vi "SaveFile.vi"(6 "Logging file refnum in":refnum<file>, 7 "Threshold Exceeded?":bool, 8 "Error in":errorcluster, 9 "Sound format":T2, 10 "Filtered Data":waveform(dbl)[](array[waveform]), 11 "Sound file refnum in":T1) -> (0 "Error out":errorcluster, 3 "Sound file refnum out":T1, 4 "Logging file refnum out":refnum<file>)   [LabVIEW 2019]
uses:
  <vilib>/sound2/lvsound2.llb/Sound File Refnum.ctl
  <vilib>/sound2/lvsound2.llb/Sound File Write Open.vi
  <vilib>/sound2/lvsound2.llb/Sound File Write (DBL).vi
  <vilib>/sound2/lvsound2.llb/Sound Data Format.ctl
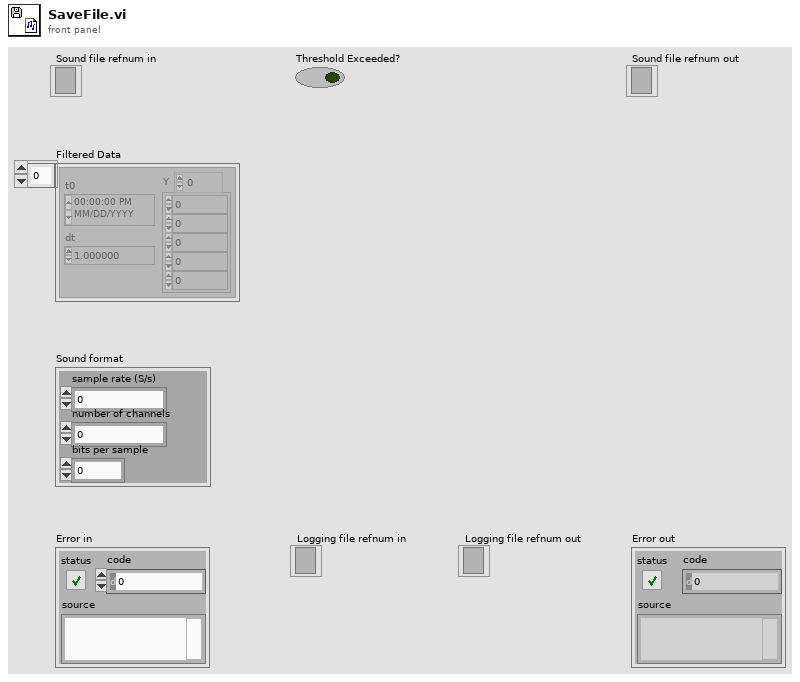
[diagram p1: front panel]
types:
  T1 = typedef "Sound File Refnum.ctl" = refnum<file>
  T2 = typedef "Sound Data Format.ctl" = cluster{"sample rate (S/s)":dbl, "number of channels":i32, "bits per sample":i32}
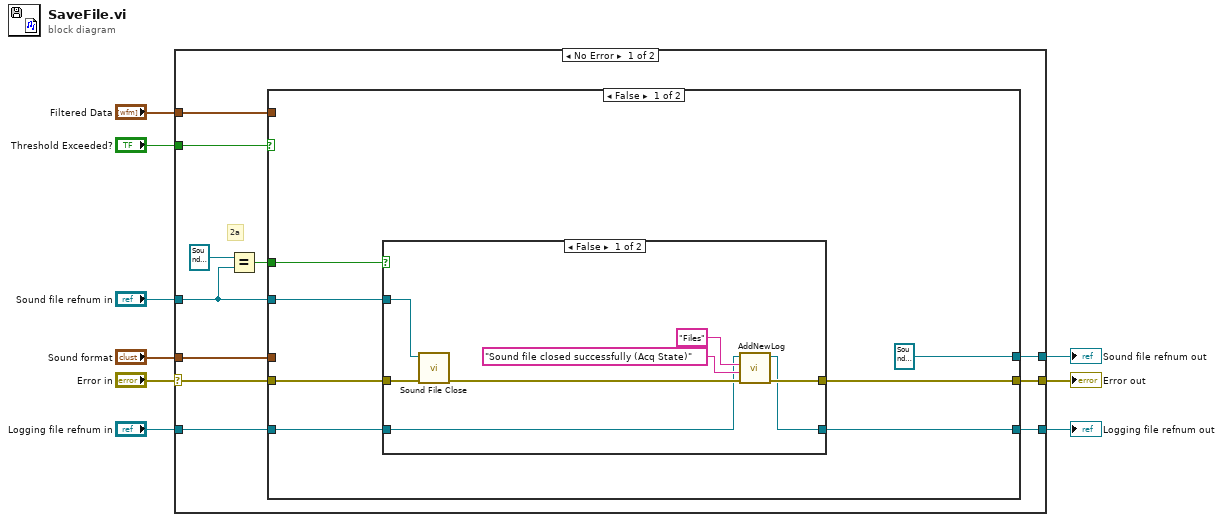
[diagram p0: block diagram]
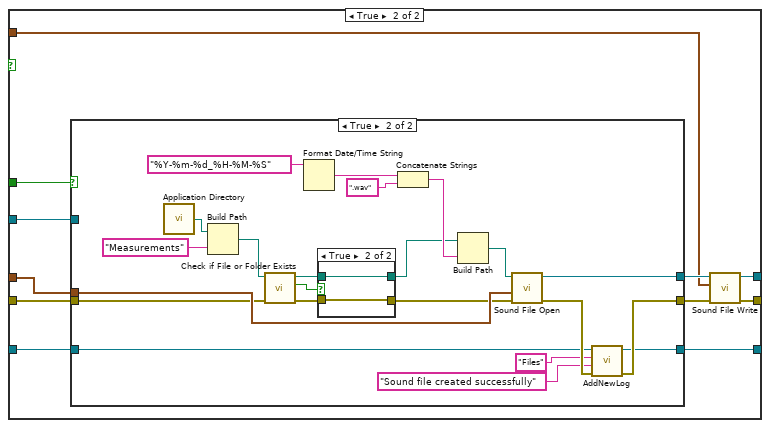
[diagram p3: hidden frame]
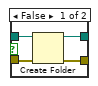
[diagram p5: hidden frame]
diagram:
  n1 = case shown="No Error" "Error in" {
    selector: "Error in" -> [w12 w82]
    tunnel: "Threshold Exceeded?" -> [w20 _]
    tunnel: "Filtered Data" -> [w19 _]
    tunnel: "Sound format" -> [w18 _]
    tunnel: [w17 w82] -> w6
    tunnel: [w16 w81] -> w5
    tunnel: "Sound file refnum in" -> [w14 w81]
    tunnel: "Logging file refnum in" -> [w11 w80]
    tunnel: [w10 w80] -> w1
    frame No Error {
      # "2a"
      n2 = Equal?(x=T1 refnum ("sound file refnum out"), y=w14) -> (x = y?=w13:bool)
      n3 = case shown="False" w20 {
        tunnel: [w25 w46] -> w17
        tunnel: w18 -> [_ w45]
        tunnel: w19 -> [_ w44]
        tunnel: w12 -> [w27 w43]
        tunnel: [T1 refnum ("sound file refnum out") w42] -> w16
        tunnel: w14 -> [w26 w40]
        tunnel: w13 -> [w23 w41]
        tunnel: w11 -> [w22 w39]
        tunnel: [w21 w38] -> w10
        frame False {
          n4 = case shown="False" w23 {
            tunnel: w27 -> [w35 w37]
            tunnel: w26 -> [w34 _]
            tunnel: [w30 w37] -> w25
            tunnel: w22 -> [w29 w36]
            tunnel: [w28 w36] -> w21
            frame False {
              n5 = call <vilib>:"Sound File Close.vi"("error in (no error)"=w35, "sound file refnum"=w34) -> ("error out"=w31:errorcluster)  [unwired: 9 in]
              n6 = call "AddNewLog.vi"("error in"=w31, "Details"="Sound file closed successfully (Acq State)" ("string"), "General Info"="Files" ("string"), "Logging file refnum in"=w29) -> ("error out"=w30:errorcluster, "Logging file refnum out"=w28:refnum<file>)  [unwired: 6 in]
            }
            frame True {
            }
          }
        }
        frame True {
          n7 = case shown="True" w41 {
            tunnel: [w50 w73] -> w48
            tunnel: [w51 w56] -> w47
            tunnel: w45 -> [_ w72]
            tunnel: w43 -> [w51 w64]
            tunnel: w40 -> [w50 _]
            tunnel: w39 -> [w49 w55]
            tunnel: [w49 w54] -> w38
            frame False {
            }
            frame True {
              n8 = call <vilib>:"Application Directory.vi"() -> ("Application Directory"=w69:path)
              n9 = Build Path(base path=w69, name or relative path="Measurements") -> (appended path=w59:path)
              n10 = call <vilib>:"Check if File or Folder Exists.vi"("error in (no error)"=w64, "path"=w59) -> ("error out"=w63:errorcluster, "file or folder exists?"=w61:bool, "dup path"=w60:path)  [unwired: 7 in]
              n11 = Format Date/Time String(time format string (%c)="%Y-%m-%d_%H-%M-%S") -> (date/time string=w70:string)  [unwired: 2 in]
              n12 = case shown="True" w61 {
                tunnel: w63 -> [w77 w79]
                tunnel: [w76 w79] -> w62
                tunnel: w60 -> [w75 w78]
                tunnel: [w74 w78] -> w58
                frame False {
                  n13 = Create Folder(path (use dialog)=w75, error in=w77) -> (created path=w74:path, error out=w76:errorcluster)  [unwired: 1 in, 1 out]
                }
                frame True {
                }
              }
              n14 = Concatenate Strings(w70, ".wav" ("string")) -> (w71:string)
              n15 = Build Path(base path=w58, name or relative path=w71) -> (appended path=w65:path)
              n16 = call-poly <vilib>:"Sound File Open.vi"("error in (no error)"=w62, "sound format"=w72, "path"=w65) -> ("error out"=w57:errorcluster, "sound file refnum"=w73:T1)  [unwired: 7 in]
              n17 = call "AddNewLog.vi"("error in"=w57, "Details"="Sound file created successfully" ("string"), "General Info"="Files" ("string"), "Logging file refnum in"=w55) -> ("error out"=w56:errorcluster, "Logging file refnum out"=w54:refnum<file>)  [unwired: 6 in]
            }
          }
          n18 = call-poly <vilib>:"Sound File Write.vi"("error in (no error)"=w47, "data"=w44, "sound file refnum"=w48) -> ("error out"=w46:errorcluster, "sound file refnum out"=w42:T1)  [unwired: 7 in]
        }
      }
    }
    frame Error {
    }
  }
  "Error out" <- w6
  "Sound file refnum out" <- w5
  "Logging file refnum out" <- w1
